vi "Query Available Printers.vi"(8 "error in (no error)":errorcluster) -> (0 "error out":errorcluster, 2 "Default Printer":string, 3 "System Configured Printers":string[](array[string]))   [LabVIEW 2020]
doc: "Lists the printers available on the computer, including the default printer in LabVIEW."
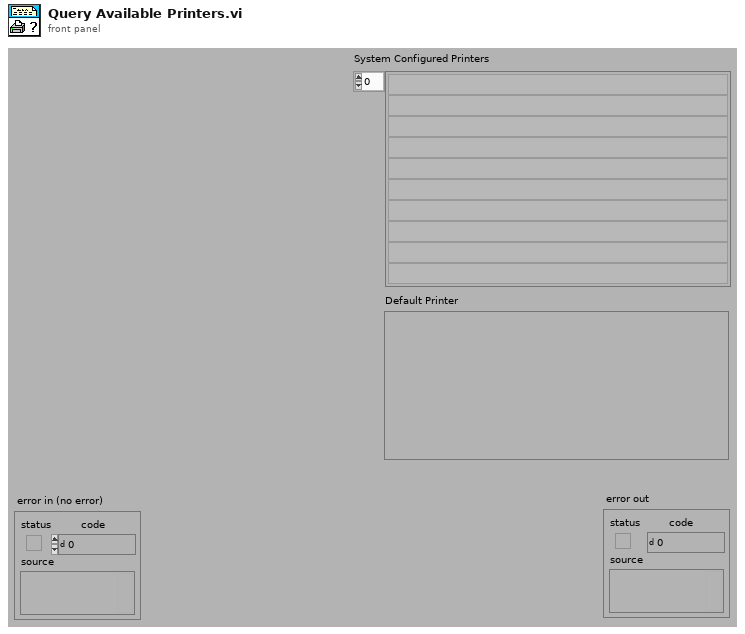
[diagram p1: front panel]
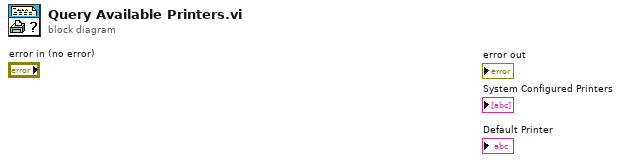
[diagram p0: block diagram]
diagram:
